vi "Autonomous Independent.vi"() -> ()   [LabVIEW 2016]
doc: "This VI is called when autonomous begins, and will automatically be terminated when autonomous ends. You can carry out timed or sensor driven robot movement independently without needing to return to the caller."
uses:
  <vilib>/Rock Robotics/WPI/DriverStation/WPI_DriverStationAllianceInfo.ctl
  <vilib>/Rock Robotics/WPI/ThirdParty/CanMotor/TalonSRX/WPI_CANTalonSRX_APIControlMode.ctl
  <vilib>/Rock Robotics/WPI/Utilities/WPI_GetSetVariantRefNum.vi
  <vilib>/Rock Robotics/Network Tables/NT Write Numeric Array.vi
  <vilib>/Rock Robotics/Network Tables/NT Read String.vi
  Robot Global Data.vi
  <vilib>/Rock Robotics/Network Tables/NT Write Boolean.vi
panel:
  in  "GearDegree":dbl
  in  "Degree Save":dbl
  out "Degree set":dbl
  # "Be sure to right-click and choose Data Operations>>Make Current Value default if you want to save the array values with the VI"
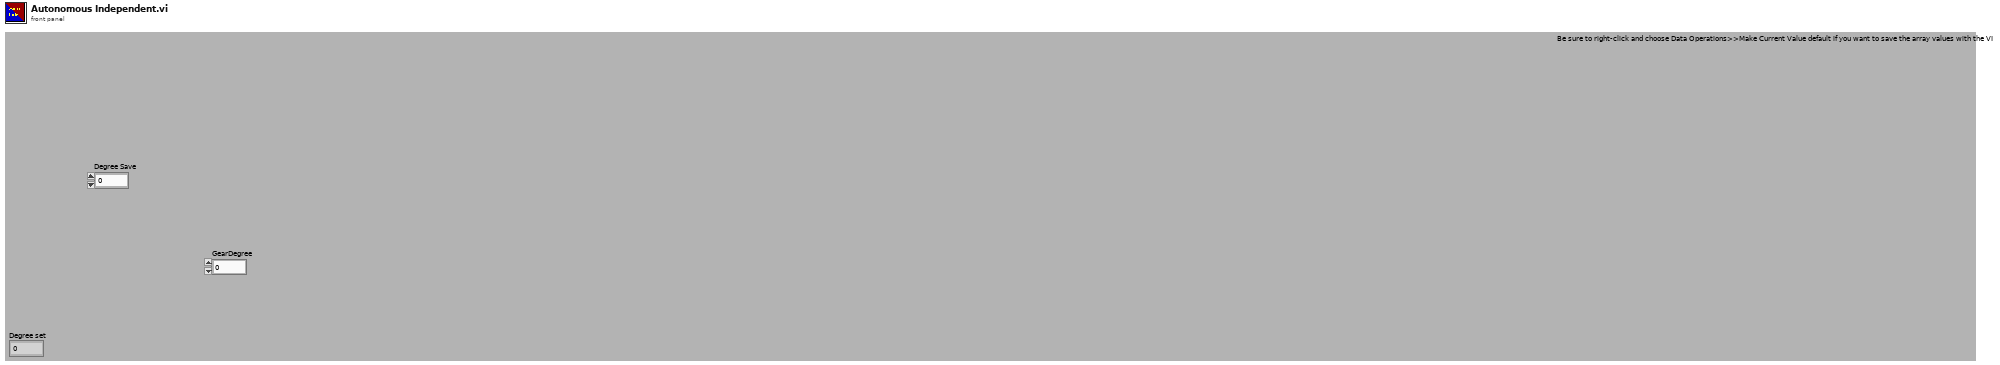
[diagram p1: front panel]
types:
  T1 = typedef "WPI_DriverStationAllianceInfo.ctl" = enum16{"Red", "Blue", "Invalid"}
  T2 = typedef "WPI_JoystickDevRef.ctl" = cluster{"Device":T3}
  T3 = typedef "WPI_JoystickDeviceEnum.ctl" = enum16{"USB 0", "USB 1", "USB 2", "USB 3", "USB 4", "USB 5"}
  T4 = typedef "WPI_CANTalonSRX_APIControlMode.ctl" = enum8{"Percent VBus", "Speed", "Position", "Slave", "Unchanged / Invalid", "Voltage Compensation", "Current", "Motion Profile", "Motion Magic"}
  T5 = typedef "WPI_MotorControlDeviceRef.ctl" = cluster{"DeviceStatus":errorcluster, "Type":T6, "PWM":cluster{"PWM Channel":T7, "DeadBand":T8}, "CAN":cluster{"Device Number":u8, "SetOutput VI Ref":variant, "GetOutput VI Ref":variant, "Enable VI Ref":variant, "Disable VI Ref":variant, "Data":variant}, "Invert":bool}
  T6 = typedef "WPI_MotorControlType.ctl" = enum16{"PWM", "CAN"}
  T7 = typedef "FPGA_DIOPWMChannel.ctl" = enum8{"PWM 0", "PWM 1", "PWM 2", "PWM 3", "PWM 4", "PWM 5", "PWM 6", "PWM 7", "PWM 8", "PWM 9", "PWM MXP 0", "PWM MXP 1", "PWM MXP 2", "PWM MXP 3", "PWM MXP 4", "PWM MXP 5", "PWM MXP 6", "PWM MXP 7", "PWM MXP 8", "PWM MXP 9", "Invalid"}
  T8 = typedef "WPI_PWMDeadband.ctl" = cluster{"Name":string, "maxPositivePwm":i32, "minPositivePwm":i32, "centerPwm":i32, "maxNegativePwm":i32, "minNegativePwm":i32, "angularRange":u16}
  T9 = typedef "WPI_GyroDevRef.ctl" = cluster{"DevStatus":errorcluster, "Analog Channel":T10, "Offset":dbl, "Gain (VoltsPerDegree/Second)":dbl, "Gyro Type":enum16{"Analog", "XRS450"}, "Handle":i32, "SPI Bus":T11, "Device Found":bool, "Sample Rate":dbl, "Calibrate On Open":bool}
  T10 = typedef "FPGA_AIChannel.ctl" = enum8{"AI 0", "AI 1", "AI 2", "AI 3", "AI MXP 0", "AI MXP 1", "AI MXP 2", "AI MXP 3", "Invalid"}
  T11 = typedef "spi_bus.ctl" = enum16{"SPI On-Board, CS0", "SPI On-Board, CS1", "SPI On-Board, CS2", "SPI On-Board, CS3", "SPI MXP", "Invalid"}
  T12 = typedef "WPI_EncoderDevRef.ctl" = cluster{"DevStatus":errorcluster, "EncoderIndex":T13, "CounterIndex":T14, "DistancePerCount":dbl, "Decoding Type":T15}
  T13 = typedef "FPGA_EncoderIdx.ctl" = enum8{"Enc 0", "Enc 1", "Enc 2", "Enc 3", "Enc 4", "Enc 5", "Enc 6", "Enc 7", "Invalid"}
  T14 = typedef "FPGA_CounterCtrSystemIndex.ctl" = enum8{"Ctr 0", "Ctr 1", "Ctr 2", "Ctr 3", "Ctr 4", "Ctr 5", "Ctr 6", "Ctr 7", "Invalid"}
  T15 = typedef "WPI_EncoderType.ctl" = enum16{"1x", "2x", "4x"}
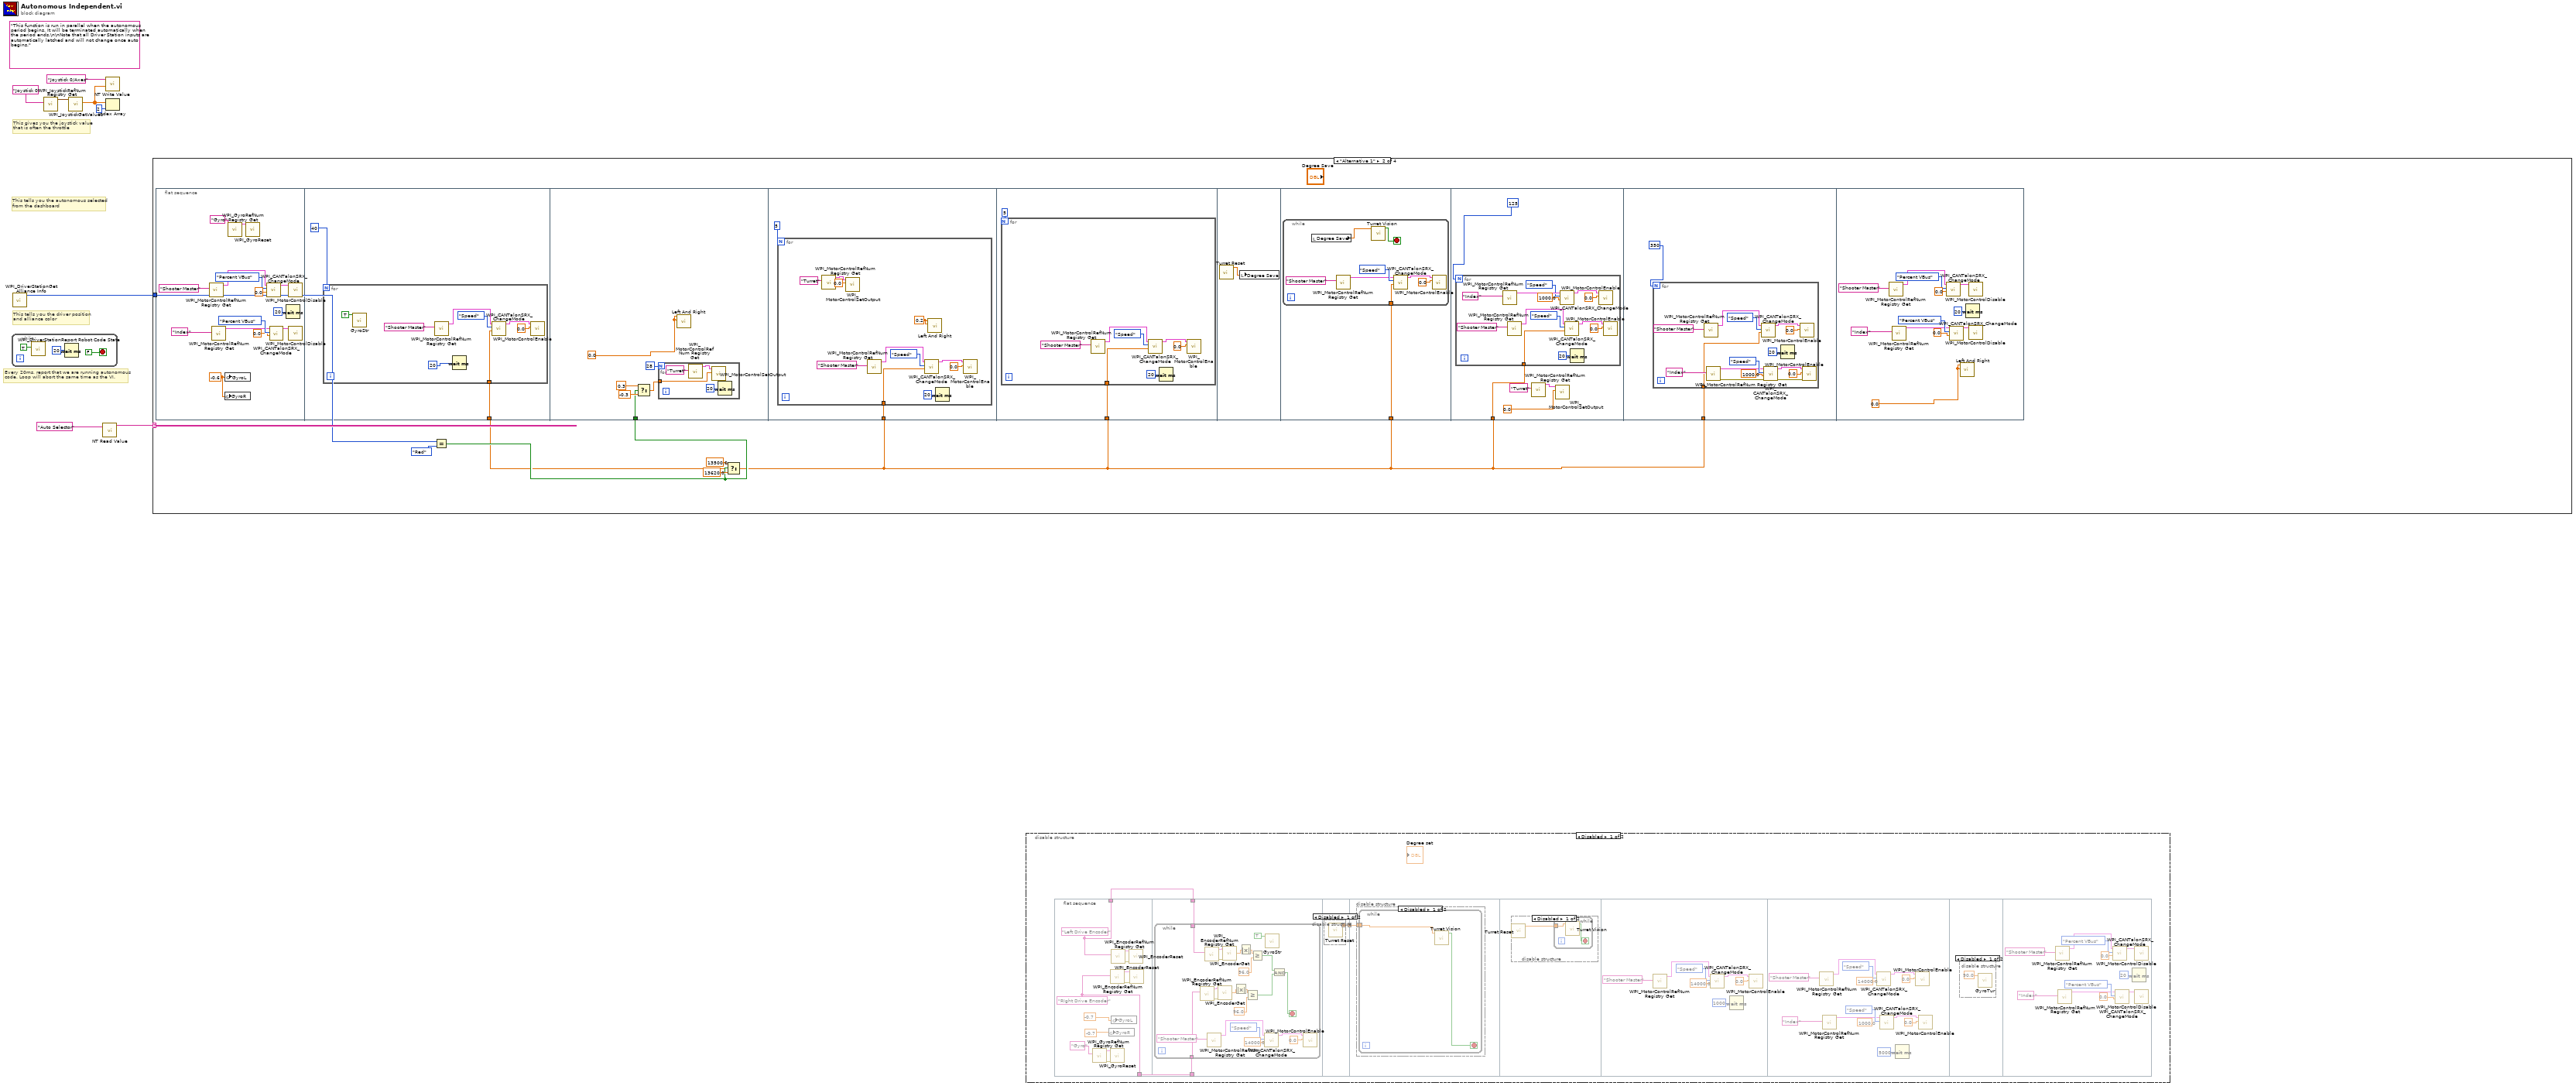
[diagram p0: block diagram]
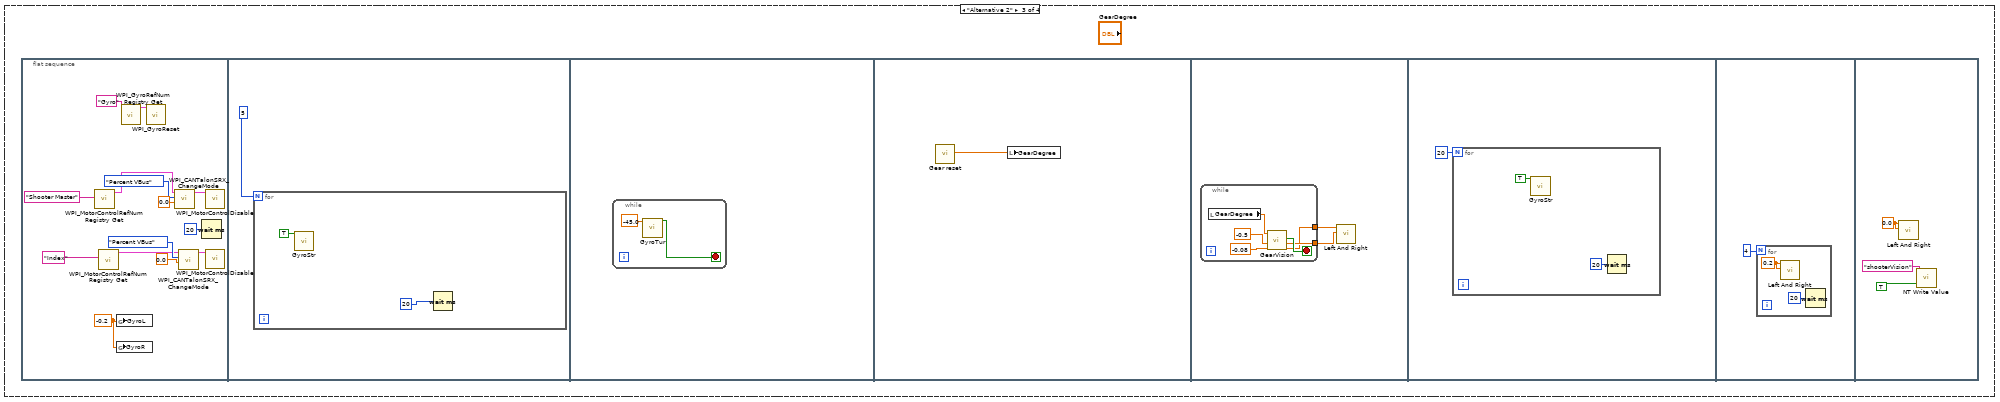
[diagram p8: hidden frame]
diagram:
  (unwired) "This function is run in parallel when the autonomous period begins. It will be terminated automatically when the period ends.\n\nNote that all Driver Station inputs are automatically latched and will not change once auto begins."
  # "This tells you the autonomous selected\nfrom the dashboard"
  # "Every 20ms, report that we are running autonomous\ncode. Loop will abort the same time as the VI."
  # "This gives you the joystick value\nthat is often the throttle"
  # "This tells you the driver position\nand alliance color"
  n1 = while {
    stop <- FALSE stop-if-true
    n2 = call <vilib>:"WPI_DriverStationReport Robot Code State.vi"("Autonomous"=TRUE) -> ()  [unwired: 10 in, 1 out]
    n3 = Wait (ms)(milliseconds to wait=u32 20) -> ()  [unwired: 1 out]
  }
  n4 = call <vilib>:"WPI_DriverStationGet Alliance Info.vi"() -> ("Alliance"=w1:T1)  [unwired: 11 out]
  n5 = call <vilib>:"WPI_JoystickRefNum Registry Get.vi"("refnum name"="Joystick 0") -> ("JoystickDevRef"=w7:T2)  [unwired: 1 in, 9 out]
  n6 = call <vilib>:"WPI_JoystickGetValues.vi"("JoystickDevRef"=w7) -> ("Axes"=w5:dbl[])  [unwired: 6 in, 4 out]
  n7 = call-poly <vilib>:"NT Read Value.vi"("Name"="Auto Selector") -> ("String"=w2:string)  [unwired: 9 in, 1 out]
  n8 = call-poly <vilib>:"NT Write Value.vi"("Numeric Array"=w5, "Name"="Joystick 0/Axes") -> ()  [unwired: 9 in, 1 out]
  n9 = Index Array(array=w5, index=2) -> ()  [unwired: 1 out]
  n10 = case shown="\"Alternative 1\"" w2 {
    tunnel: w1 -> [_ w17 _ _]
    frame Default {
      # "You can put your main auto here, or you can right-click on the case and make any\nother frame be the default case."
      # "This is the frame that will execute if no selection is made, or if it is not recognized"
    }
    frame "Alternative 1" {
      n11 = flat-sequence {
        tunnel: w12 -> [w32]
        tunnel: w13 -> [w43]
        tunnel: w12 -> [w52]
        tunnel: w12 -> [w65]
        tunnel: w12 -> [w75]
        tunnel: w12 -> [w84]
        tunnel: w12 -> [w102]
        frame #0 {
          w18 = -0.6 ("GyroL")
          n12 = call <vilib>:"WPI_MotorControlRefNum Registry Get.vi"("refnum name"="Shooter Master") -> ("MotorControlDevRef"=w27:T5)  [unwired: 9 in, 1 out]
          n13 = call <vilib>:"WPI_MotorControlRefNum Registry Get.vi"("refnum name"="Index") -> ("MotorControlDevRef"=w23:T5)  [unwired: 9 in, 1 out]
          n14 = global write "Robot Global Data.vi" "GyroR"(w18) -> ()
          n15 = global write "Robot Global Data.vi" "GyroL"(w18) -> ()
          n16 = call <vilib>:"WPI_GyroRefNum Registry Get.vi"("refnum name"="Gyro") -> ("GyroDevRef"=w31:T9)  [unwired: 9 in, 1 out]
          n17 = call <vilib>:"WPI_GyroReset.vi"("GyroDevRef"=w31) -> ()  [unwired: 9 in, 2 out]
          n18 = call <vilib>:"WPI_CANTalonSRX_ChangeMode.vi"("Output"=0.0, "Control Mode"=WPI_CANTalonSRX_APIControlMode."Percent VBus", "CAN Talon SRX Ref"=w27) -> ("CAN Talon SRX Ref"=w20:T5)  [unwired: 7 in, 1 out]
          n19 = call <vilib>:"WPI_CANTalonSRX_ChangeMode.vi"("Output"=0.0, "Control Mode"=WPI_CANTalonSRX_APIControlMode."Percent VBus", "CAN Talon SRX Ref"=w23) -> ("CAN Talon SRX Ref"=w19:T5)  [unwired: 7 in, 1 out]
          n20 = Wait (ms)(milliseconds to wait=u32 20) -> ()  [unwired: 1 out]
          n21 = call <vilib>:"WPI_MotorControlDisable.vi"("MotorControlDevRef"=w20) -> ()  [unwired: 9 in, 2 out]
          n22 = call <vilib>:"WPI_MotorControlDisable.vi"("MotorControlDevRef"=w19) -> ()  [unwired: 9 in, 2 out]
        }
        frame #1 {
          n23 = for {
            N: 40 -> [_]
            tunnel: w32 -> [w34]
            n24 = call "GyroStr.vi"("Reverse"=TRUE) -> ()  [unwired: 11 in]
            n25 = call <vilib>:"WPI_MotorControlRefNum Registry Get.vi"("refnum name"="Shooter Master") -> ("MotorControlDevRef"=w37:T5)  [unwired: 9 in, 1 out]
            n26 = Wait (ms)(milliseconds to wait=u32 20) -> ()  [unwired: 1 out]
            n27 = call <vilib>:"WPI_CANTalonSRX_ChangeMode.vi"("Output"=w34, "Control Mode"=WPI_CANTalonSRX_APIControlMode."Speed", "CAN Talon SRX Ref"=w37) -> ("CAN Talon SRX Ref"=w38:T5)  [unwired: 7 in, 1 out]
            n28 = call <vilib>:"WPI_MotorControlEnable.vi"("Encoder Initial Position"=0.0, "CAN MotorDevRef"=w38) -> ()  [unwired: 8 in, 2 out]
          }
        }
        frame #2 {
          w47 = 0.0
          n29 = Select(t=0.3, s=w43, f=-0.3) -> (s? t:f=w42:dbl)
          n30 = for {
            N: 28 -> [_]
            tunnel: w42 -> [w48]
            n31 = call <vilib>:"WPI_MotorControlRefNum Registry Get.vi"("refnum name"="Turret") -> ("MotorControlDevRef"=w50:T5)  [unwired: 9 in, 1 out]
            n32 = call <vilib>:"WPI_MotorControlSetOutput.vi"("Output"=w48, "MotorControlDevRef"=w50) -> ()  [unwired: 7 in, 3 out]
            n33 = Wait (ms)(milliseconds to wait=u32 20) -> ()  [unwired: 1 out]
          }
          n34 = call "Left And Right.vi"("Right"=w47, "Left"=w47) -> ()  [unwired: 10 in]
        }
        frame #3 {
          n35 = for {
            N: 5 -> [_]
            tunnel: w52 -> [w54]
            w58 = 0.2 ("Left")
            n36 = call <vilib>:"WPI_MotorControlRefNum Registry Get.vi"("refnum name"="Turret") -> ("MotorControlDevRef"=w56:T5)  [unwired: 9 in, 1 out]
            n37 = call <vilib>:"WPI_MotorControlSetOutput.vi"("Output"=0.0, "MotorControlDevRef"=w56) -> ()  [unwired: 7 in, 3 out]
            n38 = call <vilib>:"WPI_MotorControlRefNum Registry Get.vi"("refnum name"="Shooter Master") -> ("MotorControlDevRef"=w60:T5)  [unwired: 9 in, 1 out]
            n39 = call <vilib>:"WPI_CANTalonSRX_ChangeMode.vi"("Output"=w54, "Control Mode"=WPI_CANTalonSRX_APIControlMode."Speed", "CAN Talon SRX Ref"=w60) -> ("CAN Talon SRX Ref"=w61:T5)  [unwired: 7 in, 1 out]
            n40 = call "Left And Right.vi"("Right"=w58, "Left"=w58) -> ()  [unwired: 10 in]
            n41 = Wait (ms)(milliseconds to wait=u32 20) -> ()  [unwired: 1 out]
            n42 = call <vilib>:"WPI_MotorControlEnable.vi"("Encoder Initial Position"=0.0, "CAN MotorDevRef"=w61) -> ()  [unwired: 8 in, 2 out]
          }
        }
        frame #4 {
          n43 = for {
            N: 5 -> [_]
            tunnel: w65 -> [w67]
            n44 = call <vilib>:"WPI_MotorControlRefNum Registry Get.vi"("refnum name"="Shooter Master") -> ("MotorControlDevRef"=w69:T5)  [unwired: 9 in, 1 out]
            n45 = call <vilib>:"WPI_CANTalonSRX_ChangeMode.vi"("Output"=w67, "Control Mode"=WPI_CANTalonSRX_APIControlMode."Speed", "CAN Talon SRX Ref"=w69) -> ("CAN Talon SRX Ref"=w70:T5)  [unwired: 7 in, 1 out]
            n46 = Wait (ms)(milliseconds to wait=u32 20) -> ()  [unwired: 1 out]
            n47 = call <vilib>:"WPI_MotorControlEnable.vi"("Encoder Initial Position"=0.0, "CAN MotorDevRef"=w70) -> ()  [unwired: 8 in, 2 out]
          }
        }
        frame #5 {
          n48 = call "Turret Reset.vi"() -> ("Numeric"=w74:dbl)  [unwired: 11 in]
          n49 = local write "Degree Save"(w74) -> ()
        }
        frame #6 {
          n50 = while {
            tunnel: w75 -> [w76]
            stop <- w83 stop-if-true
            n51 = local read "Degree Save"() -> (w77:dbl)
            n52 = call <vilib>:"WPI_MotorControlRefNum Registry Get.vi"("refnum name"="Shooter Master") -> ("MotorControlDevRef"=w78:T5)  [unwired: 9 in, 1 out]
            n53 = call "Turret Vision.vi"("Degree Save"=w77) -> ("Boolean"=w83:bool)  [unwired: 10 in]
            n54 = call <vilib>:"WPI_CANTalonSRX_ChangeMode.vi"("Output"=w76, "Control Mode"=WPI_CANTalonSRX_APIControlMode."Speed", "CAN Talon SRX Ref"=w78) -> ("CAN Talon SRX Ref"=w80:T5)  [unwired: 7 in, 1 out]
            n55 = call <vilib>:"WPI_MotorControlEnable.vi"("Encoder Initial Position"=0.0, "CAN MotorDevRef"=w80) -> ()  [unwired: 8 in, 2 out]
          }
        }
        frame #7 {
          n56 = for {
            N: 125 -> [_]
            tunnel: w84 -> [w95]
            n57 = call <vilib>:"WPI_MotorControlRefNum Registry Get.vi"("refnum name"="Index") -> ("MotorControlDevRef"=w92:T5)  [unwired: 9 in, 1 out]
            n58 = call <vilib>:"WPI_MotorControlRefNum Registry Get.vi"("refnum name"="Shooter Master") -> ("MotorControlDevRef"=w97:T5)  [unwired: 9 in, 1 out]
            n59 = call <vilib>:"WPI_CANTalonSRX_ChangeMode.vi"("Output"=1000.0, "Control Mode"=WPI_CANTalonSRX_APIControlMode."Speed", "CAN Talon SRX Ref"=w92) -> ("CAN Talon SRX Ref"=w94:T5)  [unwired: 7 in, 1 out]
            n60 = call <vilib>:"WPI_CANTalonSRX_ChangeMode.vi"("Output"=w95, "Control Mode"=WPI_CANTalonSRX_APIControlMode."Speed", "CAN Talon SRX Ref"=w97) -> ("CAN Talon SRX Ref"=w98:T5)  [unwired: 7 in, 1 out]
            n61 = Wait (ms)(milliseconds to wait=u32 20) -> ()  [unwired: 1 out]
            n62 = call <vilib>:"WPI_MotorControlEnable.vi"("Encoder Initial Position"=0.0, "CAN MotorDevRef"=w94) -> ()  [unwired: 8 in, 2 out]
            n63 = call <vilib>:"WPI_MotorControlEnable.vi"("Encoder Initial Position"=0.0, "CAN MotorDevRef"=w98) -> ()  [unwired: 8 in, 2 out]
          }
          n64 = call <vilib>:"WPI_MotorControlRefNum Registry Get.vi"("refnum name"="Turret") -> ("MotorControlDevRef"=w88:T5)  [unwired: 9 in, 1 out]
          n65 = call <vilib>:"WPI_MotorControlSetOutput.vi"("Output"=0.0, "MotorControlDevRef"=w88) -> ()  [unwired: 7 in, 3 out]
        }
        frame #8 {
          n66 = for {
            N: 350 -> [_]
            tunnel: w102 -> [w104]
            n67 = call <vilib>:"WPI_MotorControlRefNum Registry Get.vi"("refnum name"="Shooter Master") -> ("MotorControlDevRef"=w114:T5)  [unwired: 9 in, 1 out]
            n68 = call <vilib>:"WPI_MotorControlRefNum Registry Get.vi"("refnum name"="Index") -> ("error out"=w108:errorcluster, "MotorControlDevRef"=w107:T5)  [unwired: 9 in]
            n69 = call <vilib>:"WPI_CANTalonSRX_ChangeMode.vi"("Output"=w104, "Control Mode"=WPI_CANTalonSRX_APIControlMode."Speed", "CAN Talon SRX Ref"=w114) -> ("CAN Talon SRX Ref"=w115:T5)  [unwired: 7 in, 1 out]
            n70 = call <vilib>:"WPI_CANTalonSRX_ChangeMode.vi"("error in (no error)"=w108, "Output"=1000.0, "Control Mode"=WPI_CANTalonSRX_APIControlMode."Speed", "CAN Talon SRX Ref"=w107) -> ("error out"=w112:errorcluster, "CAN Talon SRX Ref"=w111:T5)  [unwired: 6 in]
            n71 = Wait (ms)(milliseconds to wait=u32 20) -> ()  [unwired: 1 out]
            n72 = call <vilib>:"WPI_MotorControlEnable.vi"("Encoder Initial Position"=0.0, "CAN MotorDevRef"=w115) -> ()  [unwired: 8 in, 2 out]
            n73 = call <vilib>:"WPI_MotorControlEnable.vi"("error in (no error)"=w112, "Encoder Initial Position"=0.0, "CAN MotorDevRef"=w111) -> ()  [unwired: 7 in, 2 out]
          }
        }
        frame #9 {
          w130 = 0.0
          n74 = call <vilib>:"WPI_MotorControlRefNum Registry Get.vi"("refnum name"="Shooter Master") -> ("MotorControlDevRef"=w127:T5)  [unwired: 9 in, 1 out]
          n75 = call <vilib>:"WPI_MotorControlRefNum Registry Get.vi"("refnum name"="Index") -> ("MotorControlDevRef"=w123:T5)  [unwired: 9 in, 1 out]
          n76 = call <vilib>:"WPI_CANTalonSRX_ChangeMode.vi"("Output"=0.0, "Control Mode"=WPI_CANTalonSRX_APIControlMode."Percent VBus", "CAN Talon SRX Ref"=w127) -> ("CAN Talon SRX Ref"=w120:T5)  [unwired: 7 in, 1 out]
          n77 = call <vilib>:"WPI_CANTalonSRX_ChangeMode.vi"("Output"=0.0, "Control Mode"=WPI_CANTalonSRX_APIControlMode."Percent VBus", "CAN Talon SRX Ref"=w123) -> ("CAN Talon SRX Ref"=w119:T5)  [unwired: 7 in, 1 out]
          n78 = call "Left And Right.vi"("Right"=w130, "Left"=w130) -> ()  [unwired: 10 in]
          n79 = Wait (ms)(milliseconds to wait=u32 20) -> ()  [unwired: 1 out]
          n80 = call <vilib>:"WPI_MotorControlDisable.vi"("MotorControlDevRef"=w120) -> ()  [unwired: 9 in, 2 out]
          n81 = call <vilib>:"WPI_MotorControlDisable.vi"("MotorControlDevRef"=w119) -> ()  [unwired: 9 in, 2 out]
        }
      }
      n82 = Equal?(x=w17, y=WPI_DriverStationAllianceInfo."Red") -> (x = y?=w13:bool)
      n83 = Select(t=13500.0 ("Output"), s=w13, f=13620.0) -> (s? t:f=w12:dbl)
    }
    frame "Alternative 2" {
      n84 = flat-sequence {
        frame #0 {
          w131 = -0.2 ("GyroL")
          n85 = call <vilib>:"WPI_MotorControlRefNum Registry Get.vi"("refnum name"="Shooter Master") -> ("MotorControlDevRef"=w140:T5)  [unwired: 9 in, 1 out]
          n86 = call <vilib>:"WPI_MotorControlRefNum Registry Get.vi"("refnum name"="Index") -> ("MotorControlDevRef"=w136:T5)  [unwired: 9 in, 1 out]
          n87 = global write "Robot Global Data.vi" "GyroR"(w131) -> ()
          n88 = global write "Robot Global Data.vi" "GyroL"(w131) -> ()
          n89 = call <vilib>:"WPI_GyroRefNum Registry Get.vi"("refnum name"="Gyro") -> ("GyroDevRef"=w144:T9)  [unwired: 9 in, 1 out]
          n90 = call <vilib>:"WPI_GyroReset.vi"("GyroDevRef"=w144) -> ()  [unwired: 9 in, 2 out]
          n91 = call <vilib>:"WPI_CANTalonSRX_ChangeMode.vi"("Output"=0.0, "Control Mode"=WPI_CANTalonSRX_APIControlMode."Percent VBus", "CAN Talon SRX Ref"=w140) -> ("CAN Talon SRX Ref"=w133:T5)  [unwired: 7 in, 1 out]
          n92 = call <vilib>:"WPI_CANTalonSRX_ChangeMode.vi"("Output"=0.0, "Control Mode"=WPI_CANTalonSRX_APIControlMode."Percent VBus", "CAN Talon SRX Ref"=w136) -> ("CAN Talon SRX Ref"=w132:T5)  [unwired: 7 in, 1 out]
          n93 = Wait (ms)(milliseconds to wait=u32 20) -> ()  [unwired: 1 out]
          n94 = call <vilib>:"WPI_MotorControlDisable.vi"("MotorControlDevRef"=w133) -> ()  [unwired: 9 in, 2 out]
          n95 = call <vilib>:"WPI_MotorControlDisable.vi"("MotorControlDevRef"=w132) -> ()  [unwired: 9 in, 2 out]
        }
        frame #1 {
          n96 = for {
            N: 5 -> [_]
            n97 = call "GyroStr.vi"("Reverse"=TRUE) -> ()  [unwired: 11 in]
            n98 = Wait (ms)(milliseconds to wait=u32 20) -> ()  [unwired: 1 out]
          }
        }
        frame #2 {
          n99 = while {
            stop <- w148 stop-if-true
            n100 = call "GyroTur.vi"("Target"=-45.0) -> ("Acceptable"=w148:bool)  [unwired: 10 in]
          }
        }
        frame #3 {
          n101 = call "Gear reset.vi"() -> ("GearDegrees"=w150:dbl)  [unwired: 11 in]
          n102 = local write "GearDegree"(w150) -> ()
        }
        frame #4 {
          n103 = while {
            tunnel: [w154] -> w152
            tunnel: [w153] -> w151
            stop <- w158 stop-if-true
            n104 = local read "GearDegree"() -> (w157:dbl)
            n105 = call "GearVision.vi"("Turn"=-0.08, "Forward"=-0.5, "gearDegrees"=w157) -> ("gearVisionLeft"=w153:dbl, "gearVisionRight"=w154:dbl, "Kill"=w158:bool)  [unwired: 6 in]
          }
          n106 = call "Left And Right.vi"("Right"=w152, "Left"=w151) -> ()  [unwired: 10 in]
        }
        frame #5 {
          n107 = for {
            N: 20 -> [_]
            n108 = call "GyroStr.vi"("Reverse"=TRUE) -> ()  [unwired: 11 in]
            n109 = Wait (ms)(milliseconds to wait=u32 20) -> ()  [unwired: 1 out]
          }
        }
        frame #6 {
          n110 = for {
            N: 4 -> [_]
            w164 = 0.2 ("Left")
            n111 = call "Left And Right.vi"("Right"=w164, "Left"=w164) -> ()  [unwired: 10 in]
            n112 = Wait (ms)(milliseconds to wait=u32 20) -> ()  [unwired: 1 out]
          }
        }
        frame #7 {
          w167 = 0.0 ("Left")
          n113 = call "Left And Right.vi"("Right"=w167, "Left"=w167) -> ()  [unwired: 10 in]
          n114 = call-poly <vilib>:"NT Write Value.vi"("Boolean"=TRUE, "Name"="shooterVision") -> ()  [unwired: 9 in, 1 out]
        }
      }
    }
    frame "Your Turn" {
    }
  }
  n115 = disable-structure shown="Disabled" {
    frame Disabled {
      n116 = flat-sequence {
        tunnel: [w172] -> w169
        tunnel: [w171] -> w168
        tunnel: w169 -> [w183]
        tunnel: w168 -> [w182]
        tunnel: [w206] -> w170
        tunnel: w170 -> [w208]
        frame #0 {
          w172 = "Left Drive Encoder" ("refnum name")
          w171 = "RIght Drive Encoder" ("refnum name")
          n117 = call <vilib>:"WPI_GyroRefNum Registry Get.vi"("refnum name"="Gyro") -> ("error out"=w177:errorcluster, "GyroDevRef"=w176:T9)  [unwired: 9 in]
          n118 = global write "Robot Global Data.vi" "GyroR"(-0.7 ("GyroL")) -> ()
          n119 = call <vilib>:"WPI_GyroReset.vi"("error in"=w177, "GyroDevRef"=w176) -> ()  [unwired: 8 in, 2 out]
          n120 = call <vilib>:"WPI_EncoderRefNum Registry Get.vi"("refnum name"=w171) -> ("error out"=w181:errorcluster, "EncoderDevRef"=w180:T12)  [unwired: 9 in]
          n121 = call <vilib>:"WPI_EncoderRefNum Registry Get.vi"("refnum name"=w172) -> ("error out"=w179:errorcluster, "EncoderDevRef"=w178:T12)  [unwired: 9 in]
          n122 = global write "Robot Global Data.vi" "GyroL"(-0.7 ("GyroL")) -> ()
          n123 = call <vilib>:"WPI_EncoderReset.vi"("error in (no error)"=w179, "EncoderDevRef"=w178) -> ()  [unwired: 8 in, 2 out]
          n124 = call <vilib>:"WPI_EncoderReset.vi"("error in (no error)"=w181, "EncoderDevRef"=w180) -> ()  [unwired: 8 in, 2 out]
        }
        frame #1 {
          n125 = while {
            tunnel: w183 -> [w203]
            tunnel: w182 -> [w191]
            stop <- w194 stop-if-true
            n126 = call <vilib>:"WPI_EncoderRefNum Registry Get.vi"("refnum name"=w191) -> ("error out"=w196:errorcluster, "EncoderDevRef"=w195:T12)  [unwired: 9 in]
            n127 = call <vilib>:"WPI_EncoderRefNum Registry Get.vi"("refnum name"=w203) -> ("error out"=w204:errorcluster, "EncoderDevRef"=w205:T12)  [unwired: 9 in]
            n128 = call <vilib>:"WPI_MotorControlRefNum Registry Get.vi"("refnum name"="Shooter Master") -> ("MotorControlDevRef"=w187:T5)  [unwired: 9 in, 1 out]
            n129 = call <vilib>:"WPI_EncoderGet.vi"("error in (no error)"=w196, "EncoderDevRef"=w195) -> ("Distance"=w198:dbl)  [unwired: 4 in, 5 out]
            n130 = call <vilib>:"WPI_EncoderGet.vi"("error in (no error)"=w204, "EncoderDevRef"=w205) -> ("Distance"=w201:dbl)  [unwired: 4 in, 5 out]
            n131 = Absolute Value(x=w198) -> (abs(x)=w199:dbl)
            n132 = Absolute Value(x=w201) -> (abs(x)=w200:dbl)
            n133 = Greater Or Equal?(x=w199, y=96.0) -> (x >= y?=w192:bool)
            n134 = Greater Or Equal?(x=w200, y=96.0) -> (x >= y?=w193:bool)
            n135 = call <vilib>:"WPI_CANTalonSRX_ChangeMode.vi"("Output"=14000.0, "Control Mode"=WPI_CANTalonSRX_APIControlMode."Speed", "CAN Talon SRX Ref"=w187) -> ("CAN Talon SRX Ref"=w188:T5)  [unwired: 7 in, 1 out]
            n136 = call "GyroStr.vi"("Reverse"=TRUE) -> ()  [unwired: 11 in]
            n137 = And(x=w193, y=w192) -> (x .and. y?=w194:bool)
            n138 = call <vilib>:"WPI_MotorControlEnable.vi"("Encoder Initial Position"=0.0, "CAN MotorDevRef"=w188) -> ()  [unwired: 8 in, 2 out]
          }
        }
        frame #2 {
          n139 = disable-structure shown="Disabled" {
            disable-tunnel: [w207 _] -> w206
            frame Disabled {
              n140 = call "Turret Reset.vi"() -> ("Numeric"=w207:dbl)  [unwired: 11 in]
            }
            frame Enabled {
            }
          }
        }
        frame #3 {
          n141 = disable-structure shown="Disabled" {
            disable-tunnel: w208 -> [w209 _]
            frame Disabled {
              n142 = while {
                tunnel: w209 -> [w211]
                stop <- w210 stop-if-true
                n143 = call "Turret Vision.vi"("Degree Save"=w211) -> ("Boolean"=w210:bool)  [unwired: 10 in]
              }
            }
            frame Enabled {
            }
          }
        }
        frame #4 {
          n144 = disable-structure shown="Disabled" {
            frame Disabled {
              n145 = call "Turret Reset.vi"() -> ("Numeric"=w212:dbl)  [unwired: 11 in]
              n146 = while {
                tunnel: w212 -> [w213]
                stop <- w214 stop-if-true
                n147 = call "Turret Vision.vi"("Degree Save"=w213) -> ("Boolean"=w214:bool)  [unwired: 10 in]
              }
            }
            frame Enabled {
            }
          }
        }
        frame #5 {
          n148 = call <vilib>:"WPI_MotorControlRefNum Registry Get.vi"("refnum name"="Shooter Master") -> ("MotorControlDevRef"=w217:T5)  [unwired: 9 in, 1 out]
          n149 = call <vilib>:"WPI_CANTalonSRX_ChangeMode.vi"("Output"=14000.0, "Control Mode"=WPI_CANTalonSRX_APIControlMode."Speed", "CAN Talon SRX Ref"=w217) -> ("CAN Talon SRX Ref"=w218:T5)  [unwired: 7 in, 1 out]
          n150 = Wait (ms)(milliseconds to wait=u32 1000) -> ()  [unwired: 1 out]
          n151 = call <vilib>:"WPI_MotorControlEnable.vi"("Encoder Initial Position"=0.0, "CAN MotorDevRef"=w218) -> ()  [unwired: 8 in, 2 out]
        }
        frame #6 {
          (unwired) 1000.0 ("Output")
          n152 = call <vilib>:"WPI_MotorControlRefNum Registry Get.vi"("refnum name"="Shooter Master") -> ("MotorControlDevRef"=w229:T5)  [unwired: 9 in, 1 out]
          n153 = call <vilib>:"WPI_MotorControlRefNum Registry Get.vi"("refnum name"="Index") -> ("MotorControlDevRef"=w223:T5)  [unwired: 9 in, 1 out]
          n154 = call <vilib>:"WPI_CANTalonSRX_ChangeMode.vi"("Output"=14000.0, "Control Mode"=WPI_CANTalonSRX_APIControlMode."Speed", "CAN Talon SRX Ref"=w229) -> ("CAN Talon SRX Ref"=w230:T5)  [unwired: 7 in, 1 out]
          n155 = call <vilib>:"WPI_CANTalonSRX_ChangeMode.vi"("Control Mode"=WPI_CANTalonSRX_APIControlMode."Speed", "CAN Talon SRX Ref"=w223) -> ("CAN Talon SRX Ref"=w226:T5)  [unwired: 8 in, 1 out]
          n156 = Wait (ms)(milliseconds to wait=u32 5000) -> ()  [unwired: 1 out]
          n157 = call <vilib>:"WPI_MotorControlEnable.vi"("Encoder Initial Position"=0.0, "CAN MotorDevRef"=w230) -> ()  [unwired: 8 in, 2 out]
          n158 = call <vilib>:"WPI_MotorControlEnable.vi"("Encoder Initial Position"=0.0, "CAN MotorDevRef"=w226) -> ()  [unwired: 8 in, 2 out]
        }
        frame #7 {
          n159 = disable-structure shown="Disabled" {
            frame Disabled {
              n160 = call "GyroTur.vi"("Target"=90.0) -> ()  [unwired: 10 in, 1 out]
            }
            frame Enabled {
            }
          }
        }
        frame #8 {
          n161 = call <vilib>:"WPI_MotorControlRefNum Registry Get.vi"("refnum name"="Shooter Master") -> ("MotorControlDevRef"=w243:T5)  [unwired: 9 in, 1 out]
          n162 = call <vilib>:"WPI_MotorControlRefNum Registry Get.vi"("refnum name"="Index") -> ("MotorControlDevRef"=w239:T5)  [unwired: 9 in, 1 out]
          n163 = call <vilib>:"WPI_CANTalonSRX_ChangeMode.vi"("Output"=0.0, "Control Mode"=WPI_CANTalonSRX_APIControlMode."Percent VBus", "CAN Talon SRX Ref"=w243) -> ("CAN Talon SRX Ref"=w236:T5)  [unwired: 7 in, 1 out]
          n164 = call <vilib>:"WPI_CANTalonSRX_ChangeMode.vi"("Output"=0.0, "Control Mode"=WPI_CANTalonSRX_APIControlMode."Percent VBus", "CAN Talon SRX Ref"=w239) -> ("CAN Talon SRX Ref"=w235:T5)  [unwired: 7 in, 1 out]
          n165 = Wait (ms)(milliseconds to wait=u32 20) -> ()  [unwired: 1 out]
          n166 = call <vilib>:"WPI_MotorControlDisable.vi"("MotorControlDevRef"=w236) -> ()  [unwired: 9 in, 2 out]
          n167 = call <vilib>:"WPI_MotorControlDisable.vi"("MotorControlDevRef"=w235) -> ()  [unwired: 9 in, 2 out]
        }
      }
    }
    frame Enabled {
    }
  }
